vi "SPC_get_phot_stream_info.vi"(6 "Stream Handle":i16, 8 "Error In":errorcluster, 10 "Module No":i16, 11 "DLL Path":path) -> (0 "Error Out":errorcluster, 2 "Module No":i16, 3 "DLL Path":path, 4 "Stream Handle":i16, 5 "SPC_PhotStreamInfo":T1={"FIFO Type"=4, "Stream Type"=1, "Macro Time Clock [0.1ns]"=500, "Routing Channels"=8, "What To Read"=1, "No of Files in Stream"=1, "No of Ready Files"=0, "Stream Base Name"="", "Current FIle Name"="", "1st File Number"=0, "Current File Number"=0, "No of FIFO Overruns"=0, "Stream Size"=0, "Current Offset in Stream"=0, "Offset in Current File"=0, "No of Invalid Photons"=0, "No of Read Photons"=0, "No of Read Markers 0 (Pixel)"=0, "No of Read Markers 1 (Line)"=0, "No of Read Markers 2 (Frame)"=0, "No of Read Markers 3"=0, "Start Offset of 1st Photon (DPC-230 only)"=0, "No of Buffers"=0, "No of Ready Buffers"=0, "Current Buffer Offset"=0, "Start OR Mask"=0, "Start AND Mask"=0, "Stop OR Mask"=0, "Stop AND Mask"=0, "Start Found"=0, "Stop Reached"=0, "Start Time"=0.0, "Stop Time"=0.0, "Current Time"=0.0, "Channels Present When Start Found"=0, "Channels Present When Stop Found"=0} {"Channels Present When Start Found" format="%x"; "Stop OR Mask" format="%x"; "No of Read Markers 3" format="%x"; "What To Read" format="%x"; "Stream Type" format="%x"})   [LabVIEW 2019]
doc: "The procedure fills 'stream_info' structure with the contents of DLL internal structure of the stream defined by handle 'stream_hndl'. \nProcedure returns error, if 'stream_hndl' is not the handle of the stream opened using SPC_init_phot_stream function.\nPhotStreamInfo structure is defined in the spcm_def.h file. \n\ninfo@becker-hickl.com"
uses:
  SPC_Controls/SPC_PhotStreamInfo.ctl
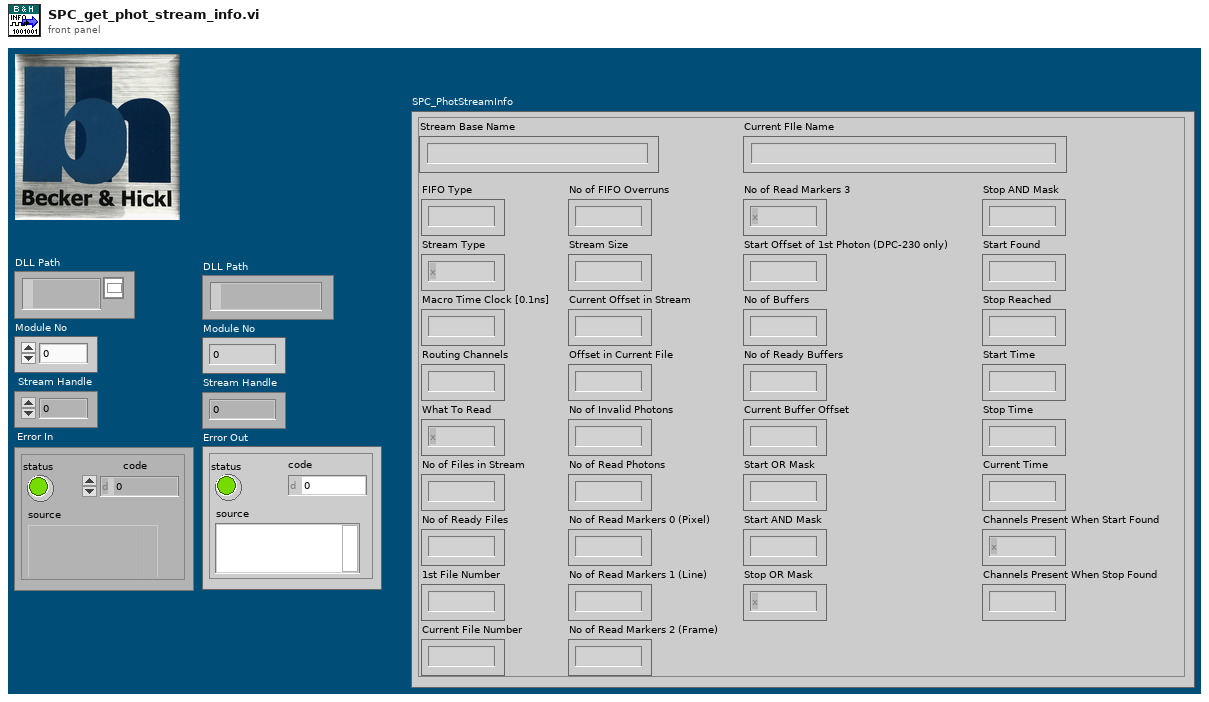
[diagram p1: front panel]
types:
  T1 = typedef "SPC_PhotStreamInfo.ctl" = cluster{"FIFO Type":i16, "Stream Type":i16, "Macro Time Clock [0.1ns]":i32, "Routing Channels":i16, "What To Read":i16, "No of Files in Stream":i16, "No of Ready Files":i16, "Stream Base Name":string, "Current FIle Name":string, "1st File Number":i16, "Current File Number":i16, "No of FIFO Overruns":i32, "Stream Size":u64, "Current Offset in Stream":u64, "Offset in Current File":u64, "No of Invalid Photons":u64, "No of Read Photons":u64, "No of Read Markers 0 (Pixel)":u64, "No of Read Markers 1 (Line)":u64, "No of Read Markers 2 (Frame)":u64, "No of Read Markers 3":u64, "Start Offset of 1st Photon (DPC-230 only)":u32, "No of Buffers":i16, "No of Ready Buffers":i16, "Current Buffer Offset":u32, "Start OR Mask":u32, "Start AND Mask":u32, "Stop OR Mask":u32, "Stop AND Mask":u32, "Start Found":i16, "Stop Reached":i16, "Start Time":dbl, "Stop Time":dbl, "Current Time":dbl, "Channels Present When Start Found":u32, "Channels Present When Stop Found":u32}
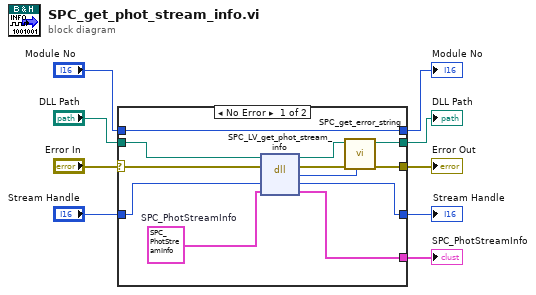
[diagram p0: block diagram]
diagram:
  n1 = case shown="No Error" "Error In" {
    selector: "Error In" -> [w20 w25]
    tunnel: [w21 w25] -> w9
    tunnel: "DLL Path" -> [w19 w24]
    tunnel: [w15 w24] -> w6
    tunnel: "Stream Handle" -> [w14 w23]
    tunnel: [w13 w23] -> w4
    tunnel: [w11 w22] -> w3
    tunnel: "Module No" -> [w11 w22]
    tunnel: [w10 _] -> w1
    frame No Error {
      w12 = T1 {"FIFO Type"=4, "Stream Type"=1, "Macro Time Clock [0.1ns]"=500, "Routing Channels"=8, "What To Read"=1, "No of Files in Stream"=1, "No of Ready Files"=0, "Stream Base Name"="", "Current FIle Name"="", "1st File Number"=0, "Current File Number"=0, "No of FIFO Overruns"=0, "Stream Size"=0, "Current Offset in Stream"=0, "Offset in Current File"=0, "No of Invalid Photons"=0, "No of Read Photons"=0, "No of Read Markers 0 (Pixel)"=0, "No of Read Markers 1 (Line)"=0, "No of Read Markers 2 (Frame)"=0, "No of Read Markers 3"=0, "Start Offset of 1st Photon (DPC-230 only)"=0, "No of Buffers"=0, "No of Ready Buffers"=0, "Current Buffer Offset"=0, "Start OR Mask"=0, "Start AND Mask"=0, "Stop OR Mask"=0, "Stop AND Mask"=0, "Start Found"=0, "Stop Reached"=0, "Start Time"=0.0, "Stop Time"=0.0, "Current Time"=0.0, "Channels Present When Start Found"=0, "Channels Present When Stop Found"=0}  # SPC_PhotStreamInfo
      n2 = dll-call lib="D:/spcm/lib/lab_view/lv10.0/spcm32.dll" fn="SPC_LV_get_phot_stream_info" label="SPC_get_phot_stream_info"(path in=w19, error in=w20, "stream_hndl"=w14, "SPC_PhotStreamInfo"=w12) -> (path out=w16:path, error out=w18:errorcluster, "return type"=w17:i16, "stream_hndl"=w13:i16, "SPC_PhotStreamInfo"=w10:T1)  [unwired: 1 in]
      n3 = call "SPC_get_error_string.vi"("ErrorID"=w17, "Error In"=w18, "DLL Path"=w16) -> ("Error Out"=w21:errorcluster, "DLL Path"=w15:path)  [unwired: 6 in, 1 out]
    }
    frame Error {
    }
  }
  "DLL Path" <- w6
  "Error Out" <- w9
  "Stream Handle" <- w4
  "Module No" <- w3
  "SPC_PhotStreamInfo" <- w1
